vi "load.vi"(8 "error in (no error)":errorcluster, 10 "Node":refnum<k20>, 11 "HP8662A_RF_Generator in":refnum<class "HP8662A_RF_Generator.lvclass">) -> (0 "error out":errorcluster, 2 "node out":refnum<k20>, 3 "HP8662A_RF_Generator out":refnum<class "HP8662A_RF_Generator.lvclass">)   [LabVIEW 2013, in "HP8662A_RF_Generator.lvclass"]
uses:
  HP8662A_RF_Generator.lvclass
  RF_Generator_settings.ctl
  HP8662A_RF_Generator.lvclass/HP8662A_RF_Generator.ctl
  Globals.vi
  <vilib>/xml/Close Reference(Node).vi
  <vilib>/xml/NI_XML.lvlib
  <resource>/objmgr/DOMUserDefRef.rc
  GPIB.lvclass
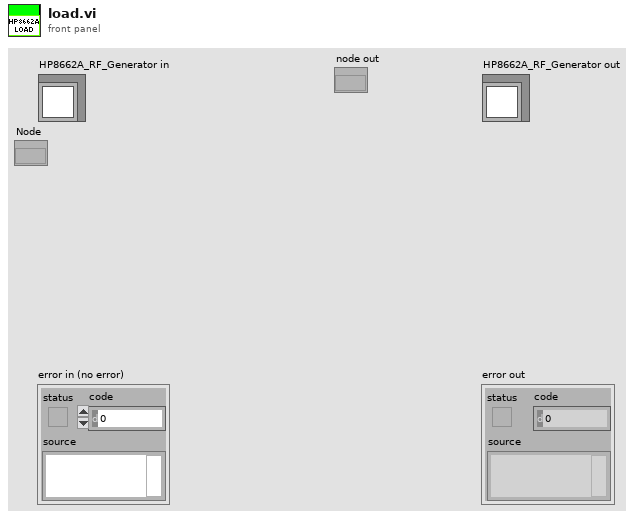
[diagram p1: front panel]
types:
  T1 = typedef "GPIB.lvclass/RF_Generator_settings.ctl" = cluster{"Enable":bool, "Description":string, "GPIB channel #":u8, "Frequency (MHz)":dbl, "Power (dBm)":dbl}
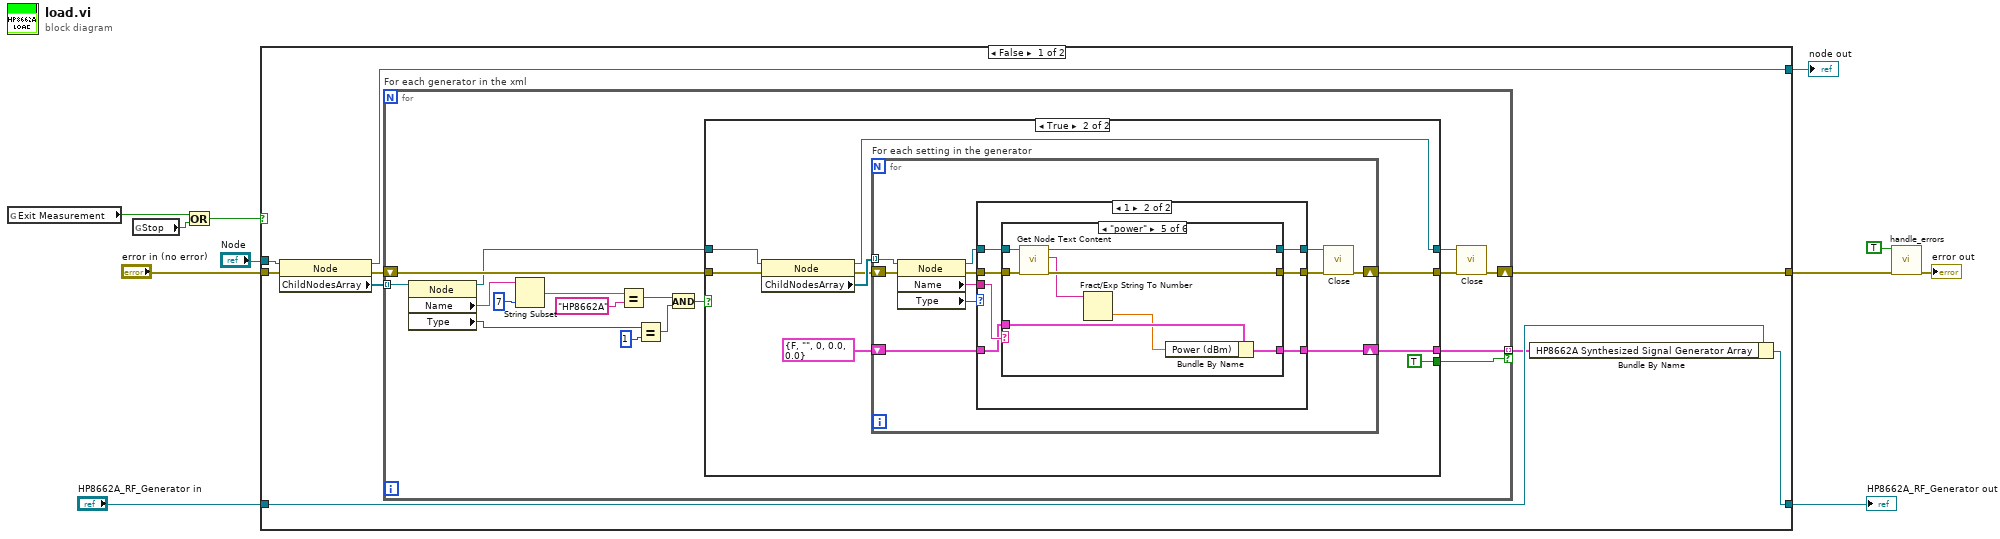
[diagram p0: block diagram]
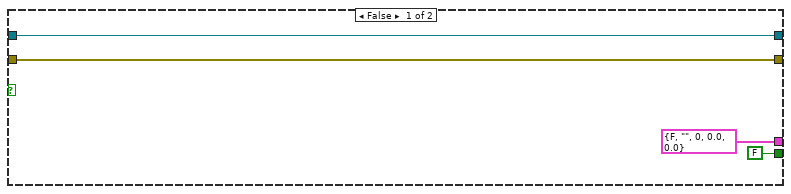
[diagram p2: hidden frame]
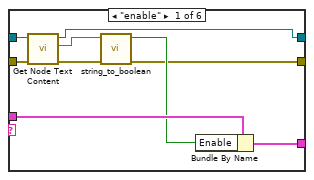
[diagram p4: hidden frame]
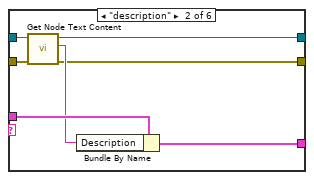
[diagram p5: hidden frame]
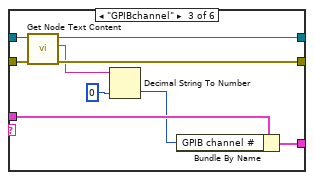
[diagram p6: hidden frame]
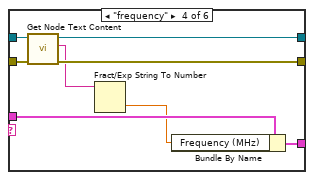
[diagram p7: hidden frame]
diagram:
  n1 = global read "Globals.vi" "Exit Measurement"() -> (w2:bool)
  n2 = global read "Globals.vi" "Stop"() -> (w3:bool)
  n3 = Or(x=w2, y=w3) -> (x .or. y?=w1:bool)
  n4 = case shown="False" w1 {
    tunnel: [w20 w117] -> w11
    tunnel: "HP8662A_RF_Generator in" -> [w19 w117]
    tunnel: "Node" -> [w17 w116]
    tunnel: "error in (no error)" -> [w16 w118]
    tunnel: [w15 w116] -> w7
    tunnel: [w12 w118] -> w6
    frame False {
      n5 = property class="Node"(reference=w17, error in=w16) -> (reference out=w15:refnum<k20>, error out=w13:errorcluster, "ChildNodesArray"=w14:refnum<k20>[])
      n6 = for "For each generator in the xml" {
        tunnel: w14 -> [w31] mode=indexing
        shift-right: [w34] -> w12
        shift-left: w13 -> [w37]
        tunnel: [w33] -> w18 mode=indexing if=w32
        n7 = property class="Node"(reference=w31) -> (reference out=w30:refnum<k20>, "Name"=w26:string, "Type"=w29:i32)  [unwired: 1 in, 1 out]
        n8 = String Subset(string=w26, length (rest)=7 ("length (rest)")) -> (substring=w24:string)  [unwired: 1 in]
        n9 = Equal?(x=w24, y="HP8662A") -> (x = y?=w22:bool)
        n10 = Equal?(x=w29, y=1) -> (x = y?=w27:bool)
        n11 = And(x=w22, y=w27) -> (x .and. y?=w21:bool)
        n12 = case shown="True" w21 {
          tunnel: w30 -> [w41 w50]
          tunnel: w37 -> [w40 w49]
          tunnel: [w41 w46] -> w36
          tunnel: [w40 w45] -> w35
          tunnel: [T1 {"Enable"=FALSE, "Description"="", "GPIB channel #"=0, "Frequency (MHz)"=0.0, "Power (dBm)"=0.0} ("Cluster") w44] -> w33
          tunnel: [FALSE TRUE] -> w32
          frame False {
          }
          frame True {
            n13 = property class="Node"(reference=w50, error in=w49) -> (reference out=w46:refnum<k20>, error out=w47:errorcluster, "ChildNodesArray"=w48:refnum<k20>[])
            n14 = for "For each setting in the generator" {
              shift-right: [w54] -> w45
              shift-left: w47 -> [w58]
              tunnel: w48 -> [w61] mode=indexing
              shift-right: [w52] -> w44
              shift-left: T1 {"Enable"=FALSE, "Description"="", "GPIB channel #"=0, "Frequency (MHz)"=0.0, "Power (dBm)"=0.0} ("Cluster") -> [w53]
              n15 = property class="Node"(reference=w61, error in=w58) -> (reference out=w56:refnum<k20>, error out=w59:errorcluster, "Name"=w60:string, "Type"=w51:i32)
              n16 = case shown="1" w51 {
                tunnel: w60 -> [_ w71]
                tunnel: w59 -> [w63 w70]
                tunnel: [w64 w69] -> w57
                tunnel: w56 -> [w64 w68]
                tunnel: [w63 w67] -> w55
                tunnel: w53 -> [w62 w66]
                tunnel: [w62 w65] -> w52
                frame Default {
                }
                frame 1 {
                  n17 = case shown="\"power\"" w71 {
                    tunnel: w70 -> [w79 w86 w95 w103 w111 w115]
                    tunnel: [w72 w81 w91 w99 w107 w115] -> w67
                    tunnel: [w76 w82 w92 w100 w108 w114] -> w69
                    tunnel: w68 -> [w80 w87 w96 w104 w112 w114]
                    tunnel: w66 -> [w78 w85 w94 w102 w110 w113]
                    tunnel: [w77 w84 w93 w101 w109 w113] -> w65
                    frame "enable" {
                      n18 = call <vilib>:"Get Node Text Content.vi"("error in (no error)"=w79, "node in"=w80) -> ("error out"=w73:errorcluster, "node text"=w75:string, "node out"=w76:refnum<k20>)  [unwired: 7 in]
                      n19 = call "string_to_boolean.vi"("error in"=w73, "string"=w75) -> ("error out"=w72:errorcluster, "boolean"=w74:bool)  [unwired: 8 in]
                      n20 = Bundle By Name(cluster=w78, "Enable"=w74) -> (w77:T1)
                    }
                    frame "description" {
                      n21 = call <vilib>:"Get Node Text Content.vi"("error in (no error)"=w86, "node in"=w87) -> ("error out"=w81:errorcluster, "node text"=w83:string, "node out"=w82:refnum<k20>)  [unwired: 7 in]
                      n22 = Bundle By Name(cluster=w85, "Description"=w83) -> (w84:T1)
                    }
                    frame "GPIBchannel" {
                      n23 = call <vilib>:"Get Node Text Content.vi"("error in (no error)"=w95, "node in"=w96) -> ("error out"=w91:errorcluster, "node text"=w90:string, "node out"=w92:refnum<k20>)  [unwired: 7 in]
                      n24 = Decimal String To Number(string=w90, default (0L)=u8 0 ("default (0 I32)")) -> (number=w89:u8)  [unwired: 1 in, 1 out]
                      n25 = Bundle By Name(cluster=w94, "GPIB channel #"=w89) -> (w93:T1)
                    }
                    frame "frequency" {
                      n26 = call <vilib>:"Get Node Text Content.vi"("error in (no error)"=w103, "node in"=w104) -> ("error out"=w99:errorcluster, "node text"=w98:string, "node out"=w100:refnum<k20>)  [unwired: 7 in]
                      n27 = Fract/Exp String To Number(string=w98) -> (number=w97:dbl)  [unwired: 3 in, 1 out]
                      n28 = Bundle By Name(cluster=w102, "Frequency (MHz)"=w97) -> (w101:T1)
                    }
                    frame "power" {
                      n29 = call <vilib>:"Get Node Text Content.vi"("error in (no error)"=w111, "node in"=w112) -> ("error out"=w107:errorcluster, "node text"=w106:string, "node out"=w108:refnum<k20>)  [unwired: 7 in]
                      n30 = Fract/Exp String To Number(string=w106) -> (number=w105:dbl)  [unwired: 3 in, 1 out]
                      n31 = Bundle By Name(cluster=w110, "Power (dBm)"=w105) -> (w109:T1)
                    }
                    frame Default {
                    }
                  }
                }
              }
              n32 = call-poly <vilib>:"Close.vi"("error in (no error)"=w55, "node"=w57) -> ("error out"=w54:errorcluster)  [unwired: 7 in]
            }
          }
        }
        n33 = call-poly <vilib>:"Close.vi"("error in (no error)"=w35, "node"=w36) -> ("error out"=w34:errorcluster)  [unwired: 7 in]
      }
      n34 = Bundle By Name(cluster=w19, "HP8662A Synthesized Signal Generator Array"=w18) -> (w20:refnum<class "HP8662A_RF_Generator.lvclass">)
    }
    frame True {
    }
  }
  "HP8662A_RF_Generator out" <- w11
  "node out" <- w7
  n35 = call "handle_errors.vi"("Exit Operation"=TRUE, "error in (no error)"=w6) -> ("error out"=→"error out":errorcluster)  [unwired: 13 in]
